vi "Subvi trigger AO DO.vi"(9 "Manual trigger":bool) -> ()   [LabVIEW 2017]
uses:
  <vilib>/Platform/TimedLoop/XDataNode/wakeup.ctl
  <vilib>/Platform/TimedLoop/XDataNode/XDNodeRunTimeDep.lvlib
  <vilib>/Platform/TimedLoop/XDataNode/nitl_modes.ctl
  <vilib>/Platform/TimedLoop/XDataNode/timing_clust.ctl
  <vilib>/Platform/TimedLoop/XDataNode/XDataNode.xnode
  GV trigger delay.vi
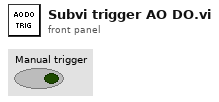
[diagram p1: front panel]
types:
  T1 = typedef "XDNodeRunTimeDep.lvlib/timing_clust.ctl" = cluster{"Expected End [f-1]":u64, "Actual End [f-1]":u64, "Finished Late? [f-1]":bool, "Expected End [i-1]":u64, "Actual End [i-1]":u64, "Finished Late? [i-1]":bool, "Expected Start [i]":u64, "Actual Start [i]":u64, "Expected Start [f]":u64, "Actual Start [f]":u64, "Source Name":string, "Structure Name":string, "Period":i64, "Deadline":i64, "Offset":i64, "Start":i64, "Priority":i32, "Timeout":i32, "Mode":T2, "Wakeup Reason":T3, "Error":errorcluster, "Source Type":string, "Secondary Source Type":string, "Global End Time":u64, "Global Start Time":u64, "Frame Duration":u64, "Iteration Duration":u64, "Assigned CPU":i32, "I/O Scan Engine Mode":u32}
  T2 = typedef "XDNodeRunTimeDep.lvlib/nitl_modes.ctl" = enum32{"No Change", "Process missed periods, maintain original phase", "Discard missed periods, maintain original phase", "Process missed periods, ignore original phase", "Discard missed periods, ignore original phase"}
  T3 = typedef "XDNodeRunTimeDep.lvlib/wakeup.ctl" = enum32{"Normal", "Aborted", "Asynchronous wakeup", "Timing source error", "Timed loop error", "Timeout"}
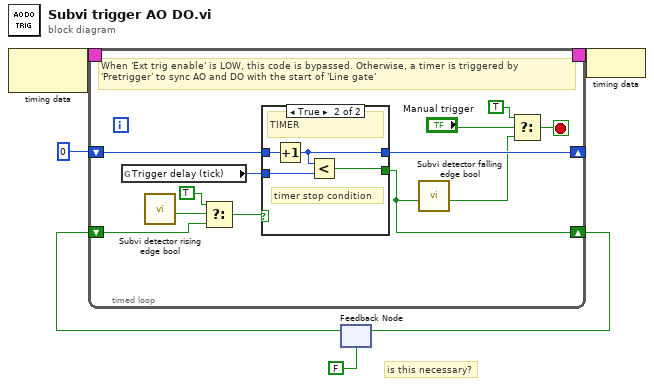
[diagram p0: block diagram]
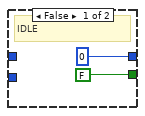
[diagram p2: hidden frame]
diagram:
  # "is this necessary?"
  n1 = node-c288() -> (w6:T1)  [unwired: 1 in]
  n2 = feedback #1(FALSE) -> (w2:bool)
  n3 = timed-loop {
    timing: w6 -> [_]
    timing-out: [_] -> w5
    shift-right: [w9] -> w1
    shift-left: w2 -> [w12]
    shift-right: [w15] -> _
    shift-left: u16 0 -> [w14]
    stop <- w10 stop-if-true
    # "When 'Ext trig enable' is LOW, this code is bypassed. Otherwise, a timer is triggered by\n'Pretrigger' to sync AO and DO with the start of 'Line gate'"
    n4 = global read "GV trigger delay.vi" "Trigger delay (tick)"() -> (w13:u16)
    n5 = call "Subvi detector rising edge bool.vi"() -> ("Output"=w16:bool)  [unwired: 11 in]
    n6 = Select(t=TRUE, s=w16, f=w12) -> (s? t:f=w17:bool)
    n7 = case shown="True" w17 {
      tunnel: [FALSE w22] -> w9
      tunnel: [u16 0 w23] -> w15
      tunnel: w14 -> [_ w24]
      tunnel: w13 -> [_ w21]
      frame False {
        # "IDLE"
      }
      frame True {
        # "timer stop condition"
        # "TIMER"
        n8 = Increment(x=w24) -> (x+1=w23:u16)
        n9 = Less?(x=w23, y=w21) -> (x < y?=w22:bool)
      }
    }
    n10 = call "Subvi detector falling edge bool.vi"("Input"=w9) -> ("Output"=w7:bool)  [unwired: 10 in]
    n11 = Select(t=TRUE, s="Manual trigger", f=w7) -> (s? t:f=w10:bool)
  }
  n12 = feedback-in #1(w1) -> ()
  n13 = node-c288(w5) -> ()
